vi "Update From Result.vi"(8 "error in (no error)":errorcluster, 10 "Result Row":refnum<class "Result Row.lvclass">, 11 "User in":refnum<class "User.lvclass">) -> (0 "error out":errorcluster, 3 "User out":refnum<class "User.lvclass">)   [LabVIEW 2022 SP3]
uses:
  User.lvclass
  Conditum/Result Row/Result Row.lvclass
  User.lvclass/User.ctl
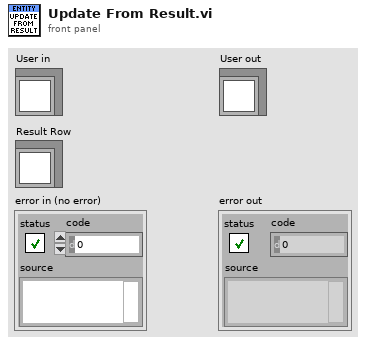
[diagram p1: front panel]
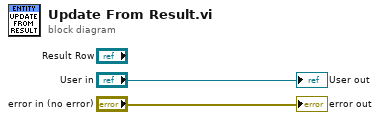
[diagram p0: block diagram]
diagram:
  "error out" <- "error in (no error)"
  "User out" <- "User in"
